vi "InitAppearance.vi"(7 "Col Array Ref in":refnum<vi>, 8 "error in (no error)":errorcluster, 9 "Table Ref in":refnum<vi>, 10 "Col #":i32, 11 "SingleValCol in":refnum<class "SingleValCol.lvclass">) -> (0 "error out":errorcluster, 1 "Table Ref out":refnum<vi>, 3 "SingleValCol out":refnum<class "SingleValCol.lvclass">, 4 "Needs 2nd pass":bool)   [LabVIEW 2013, in "SingleValCol.lvclass"]
uses:
  SingleValCol.lvclass
  <vilib>/Utility/miscctls.llb/LVRowAndColumnTypeDef.ctl
  Column/Column.lvclass/Column.ctl
  Globals/DisabledColorGlobal.vi
  Column/Column.lvclass
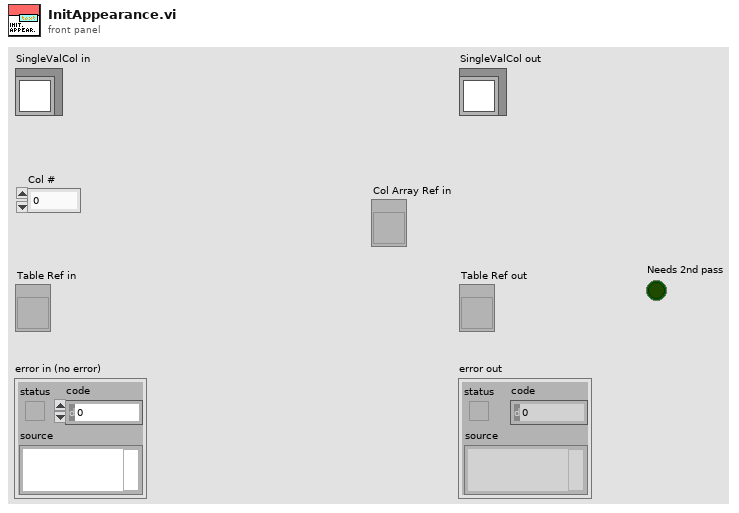
[diagram p1: front panel]
types:
  T1 = typedef "LVRowAndColumnTypeDef.ctl" = cluster{"Row":i32, "Column":i32}
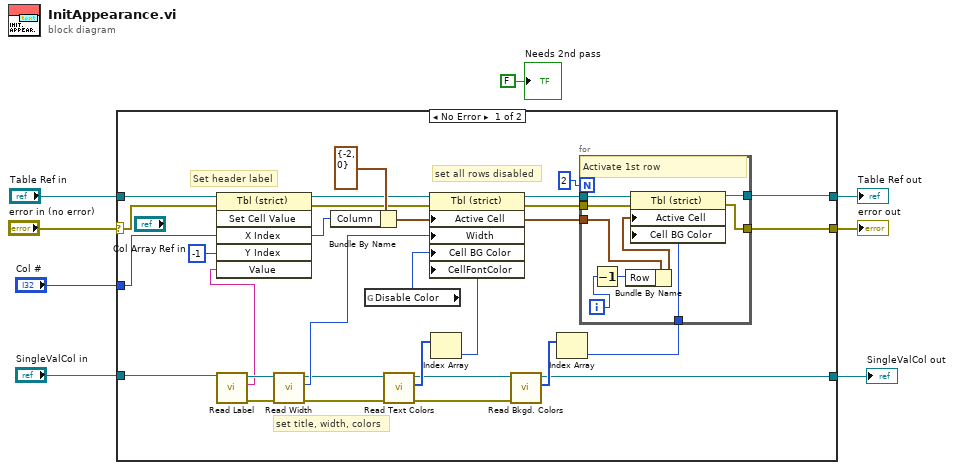
[diagram p0: block diagram]
diagram:
  n1 = case shown="No Error" "error in (no error)" {
    selector: "error in (no error)" -> [w25 w46]
    tunnel: [w19 w46] -> w7
    tunnel: [w9 w48] -> w8
    tunnel: "SingleValCol in" -> [w23 w48]
    tunnel: "Table Ref in" -> [w26 w47]
    tunnel: [w21 w47] -> w6
    tunnel: "Col #" -> [w24 _]
    frame No Error {
      # "Set header label"
      # "set title, width, colors"
      # "set all rows disabled"
      n2 = call "Read Label.vi"("Column in"=w23) -> ("error out"=w14:errorcluster, "Label"=w35:string, "Column out"=w36:refnum<class "SingleValCol.lvclass">)  [unwired: 8 in]
      n3 = invoke on="Invoke Node" class="Tbl (strict)" method="Set Cell Value"(reference=w26, error in=w25, "X Index"=w24, "Y Index"=-1 ("X Index"), "Value"=w35) -> (reference out=w28:refnum<vi>, error out=w27:errorcluster)  [unwired: 1 in, 4 out]
      n4 = call "Read Width.vi"("error in (no error)"=w14, "Column in"=w36) -> ("error out"=w13:errorcluster, "Width"=w29:u32, "Column out"=w12:refnum<class "SingleValCol.lvclass">)  [unwired: 7 in]
      n5 = Bundle By Name(cluster=T1 {"Row"=-2, "Column"=0} ("RowAndCollumn"), "Column"=w24) -> (w16:T1)
      n6 = global read "DisabledColorGlobal.vi" "Disable Color"() -> (w17:u32)
      n7 = call "Read Text Colors.vi"("error in (no error)"=w13, "Column in"=w12) -> ("error out"=w10:errorcluster, "Text Colors"=w32:u32[], "Column out"=w11:refnum<class "SingleValCol.lvclass">)  [unwired: 7 in]
      n8 = Index Array(array=w32) -> (element=w31:u32)  [unwired: 1 in]
      n9 = property class="Tbl (strict)"(reference=w28, error in=w27, "Active Cell"=w16, "Width"=w29, "Cell BG Color"=w17, "CellFontColor"=w31) -> (reference out=w22:refnum<vi>, error out=w20:errorcluster)
      n10 = call "Read Bkgd. Colors.vi"("error in (no error)"=w10, "Column in"=w11) -> ("Bkgd. Colors"=w30:u32[], "Column out"=w9:refnum<class "SingleValCol.lvclass">)  [unwired: 7 in, 1 out]
      n11 = Index Array(array=w30) -> (element=w18:u32)  [unwired: 1 in]
      n12 = for {
        N: 2 -> [_]
        tunnel: w22 -> [w45]
        tunnel: [w44] -> w21
        tunnel: w20 -> [w43]
        tunnel: [w42] -> w19
        tunnel: w18 -> [w41]
        tunnel: w16 -> [w39]
        i -> [w37]
        # "Activate 1st row"
        n13 = Decrement(x=w37) -> (x-1=w38:i32)
        n14 = Bundle By Name(cluster=w39, "Row"=w38) -> (w40:T1)
        n15 = property class="Tbl (strict)"(reference=w45, error in=w43, "Active Cell"=w40, "Cell BG Color"=w41) -> (reference out=w44:refnum<vi>, error out=w42:errorcluster)
      }
    }
    frame Error {
    }
  }
  "error out" <- w7
  "SingleValCol out" <- w8
  "Table Ref out" <- w6
  "Needs 2nd pass" <- FALSE ("Needs 2nd pass")
